vi "ChartTesting.vi"() -> ()   [LabVIEW 2014]
panel:
  out "overflow":bool
  out "count":i32
  out "Dev":i32[](array[numeric])
  out "Colors 5":u32[](array[colorbox])=[11796480, 37103, 40712, 16770816, 11796658, 4210752, 9567230, 16741120, 750336, 786687, 7565056, 16777222, 11121611, 2817859, 16728723, 16711686, 4340736]
  out "Percent % 5":dbl[](array[numeric]) format="%.2f"
  out "Connected devices":picture
  out "String 15":string
  out "String 14":string
  out "Percent % 4":dbl[](array[numeric]) format="%.2f"
  out "Colors 4":u32[](array[colorbox])=[11796480, 37103, 40712, 16770816, 11796658, 4210752]
  out "Pie Chart All data\nto user data":picture
  out "String 13":string
  out "String 12":string
  out "String 11":string
  out "String 10":string
  out "String 9":string
  out "String 8":string
  out "String 7":string
  out "String 6":string
  out "String 5":string
  out "String 4":string
  out "Percent % 3":dbl[](array[numeric]) format="%.2f"
  out "Colors 3":u32[](array[colorbox])=[11796480, 37103, 40712, 16770816, 11796658, 4210752, 15517151]
  out "Pie Chart All Tansactions":picture
  out "String 3":string
  out "String 2":string
  out "String":string
  out "Percent % 2":dbl[](array[numeric]) format="%.2f"
  out "Pie Chart Bandwidth \nof Frame":picture
  out "Colors 2":u32[](array[colorbox])=[11796480, 37103, 40712, 16770816, 11796658, 4210752]
  out "Colors":u32[](array[colorbox])=[65535, 16711935, 16776960, 16770816, 11796658, 4210752]
  out "Percent %":dbl[](array[numeric]) format="%.2f"
  out "Pie Chart Transactions: In - Out - Nak":picture
  out "Frame":cluster{i32[], i32[]}[](graph)
  out "In":cluster{i32[], i32[]}(graph)
  out "Nak":cluster{i32[], i32[]}(graph)
  out "Out":cluster{i32[], i32[]}(graph)
  in  "stop":bool
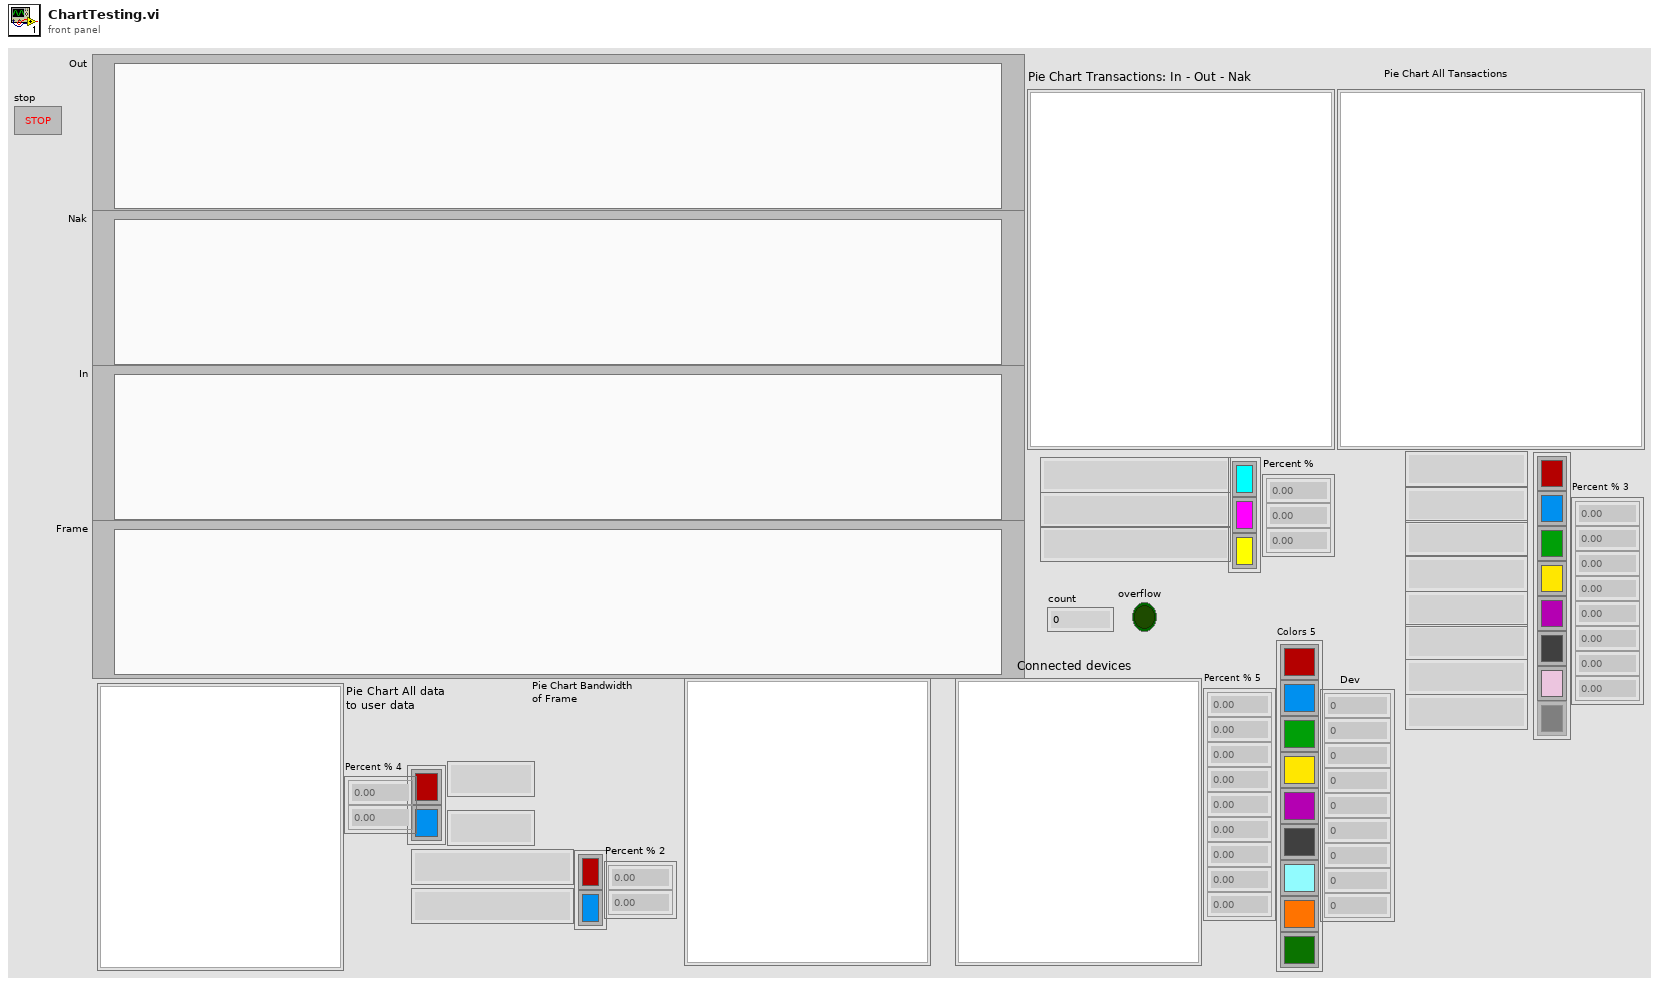
[diagram p1: front panel]
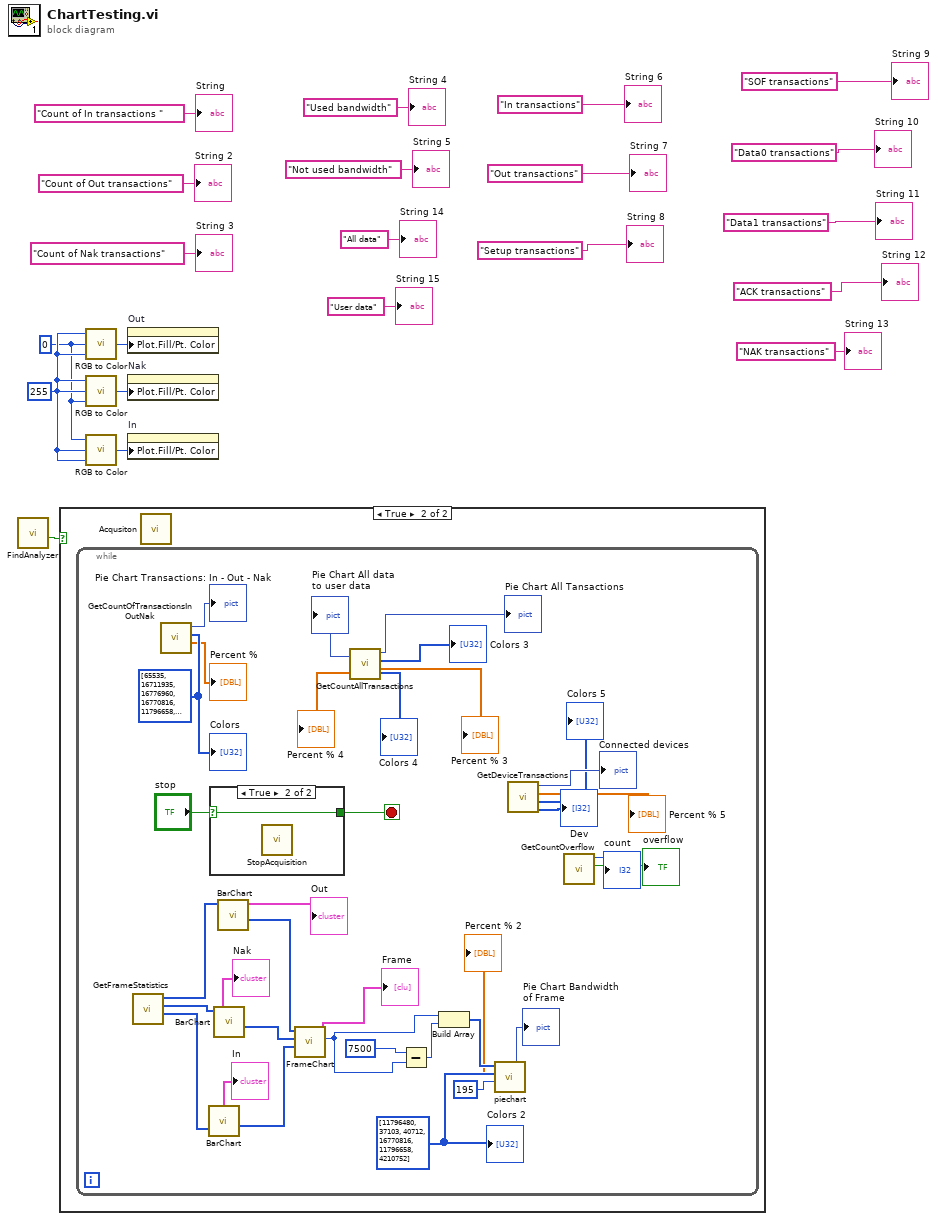
[diagram p0: block diagram]
diagram:
  w18 = u8 255
  w17 = u8 0
  n1 = call "FindAnalyzer.vi"() -> ("IsFound"=w21:bool)  [unwired: 9 in, 2 out]
  n2 = case shown="True" w21 {
    frame False {
    }
    frame True {
      n3 = while {
        stop <- w42 stop-if-true
        w37 = u32[] [11796480, 37103, 40712, 16770816, 11796658, 4210752] ("Colors")
        w44 = u32[] [65535, 16711935, 16776960, 16770816, 11796658, 4210752] ("Colors")
        n4 = call "GetFrameStatistics.vi"() -> ("FrameIn"=w49:u8[], "FrameNak"=w50:u8[], "FrameOut"=w51:u8[])  [unwired: 8 in, 1 out]
        n5 = call "GetCountOfTransactionsInOutNak.vi"("Colors"=w44) -> ("Percent %"=→"Percent %":dbl[], "Pie Chart Transactions: In - Out- Nak"=→"Pie Chart Transactions: In - Out - Nak":picture)  [unwired: 9 in]
        n6 = call "BarChart.vi"("Array Frame Statistic"=w49) -> ("X frame matrix"=w46:u8[], "XY Graph"=→"In":cluster{i32[], i32[]})  [unwired: 9 in]
        n7 = case shown="True" "stop" {
          selector: "stop" -> [_ w57]
          tunnel: [_ w57] -> w42
          frame False {
          }
          frame True {
            n8 = call "StopAcquisition.vi"() -> ()  [unwired: 10 in, 2 out]
          }
        }
        n9 = call "BarChart.vi"("Array Frame Statistic"=w50) -> ("X frame matrix"=w47:u8[], "XY Graph"=→"Nak":cluster{i32[], i32[]})  [unwired: 9 in]
        n10 = call "BarChart.vi"("Array Frame Statistic"=w51) -> ("X frame matrix"=w48:u8[], "XY Graph"=→"Out":cluster{i32[], i32[]})  [unwired: 9 in]
        n11 = call "FrameChart.vi"("Frame IN"=w46, "Frame NAK"=w47, "Frame Out"=w48) -> ("CountOfTransactionsInFrame"=w38:i32, "Frame"=→"Frame":cluster{i32[], i32[]}[])  [unwired: 7 in]
        n12 = call "GetCountAllTransactions.vi"() -> ("Percent %"=→"Percent % 3":dbl[], "Colors"=→"Colors 3":u32[], "Pie Chart All Transactions"=→"Pie Chart All Tansactions":picture, "Colors 2"=→"Colors 4":u32[], "Pie Chart All data to user data"=→"Pie Chart All data\nto user data":picture, "Percent % 2"=→"Percent % 4":dbl[])  [unwired: 6 in]
        n13 = Subtract(x=7500, y=w38) -> (x-y=w39:i32)
        n14 = Build Array(w38, w39) -> (w41:i32[])
        n15 = call "piechart.vi"("Pie Chart Size"=i16 195, "Colors"=w37, "Values"=w41) -> ("Percent %"=→"Percent % 2":dbl[], "Pie Chart"=→"Pie Chart Bandwidth \nof Frame":picture)  [unwired: 5 in]
        n16 = call "GetDeviceTransactions.vi"() -> ("Dev"=→"Dev":i32[], "Colors"=→"Colors 5":u32[], "Percent %"=→"Percent % 5":dbl[], "Pie Chart"=→"Connected devices":picture)  [unwired: 8 in]
        n17 = call "GetCountOverflow.vi"() -> ("overflow"=→"overflow":bool, "count"=→"count":i32)  [unwired: 10 in]
        "Colors" <- w44
        "Colors 2" <- w37
      }
      n18 = call "Acqusiton.vi"() -> ()  [unwired: 10 in, 2 out]
    }
  }
  n19 = call <vilib>:"RGB to Color.vi"("B"=w18, "G"=w17, "R"=w18) -> ("Color"=w16:u32)
  n20 = call <vilib>:"RGB to Color.vi"("B"=w17, "G"=w18, "R"=w18) -> ("Color"=w20:u32)
  n21 = call <vilib>:"RGB to Color.vi"("B"=w18, "G"=w18, "R"=w17) -> ("Color"=w19:u32)
  n22 = property on="Out" class="XYGraph (strict)"("Plot.Fill/Pt. Color"=w16) -> ()  [unwired: 2 in, 2 out]
  n23 = property on="Nak" class="XYGraph (strict)"("Plot.Fill/Pt. Color"=w20) -> ()  [unwired: 2 in, 2 out]
  n24 = property on="In" class="XYGraph (strict)"("Plot.Fill/Pt. Color"=w19) -> ()  [unwired: 2 in, 2 out]
  "String" <- "Count of In transactions " ("String")
  "String 2" <- "Count of Out transactions" ("String 2")
  "String 3" <- "Count of Nak transactions" ("String 3")
  "String 4" <- "Used bandwidth" ("String 4")
  "String 5" <- "Not used bandwidth" ("String 5")
  "String 6" <- "In transactions" ("String 6")
  "String 7" <- "Out transactions" ("String 7")
  "String 8" <- "Setup transactions" ("String 8")
  "String 9" <- "SOF transactions" ("String 9")
  "String 10" <- "Data0 transactions" ("String 10")
  "String 11" <- "Data1 transactions" ("String 11")
  "String 12" <- "ACK transactions" ("String 12")
  "String 13" <- "NAK transactions" ("String 13")
  "String 14" <- "All data" ("String 14")
  "String 15" <- "User data" ("String 15")
